vi "cqtDDSdllOpen.vi"   [LabVIEW 2009, in "run.lvlib"]
uses:
  run.lvlib
  C:/Program Files/National Instruments/LabVIEW 2009/instr.lib/CQT_DDS/DDSLibrary/20111109/CQTAD9958.dll
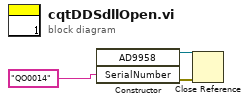
[diagram p0: block diagram]
diagram:
  n1 = constructor class="AD9958"("SerialNumber"="QO0014") -> (reference out=w1:refnum<k24>, error out=w3:errorcluster)  [unwired: 3 in, 2 out]
  n2 = Close Reference(reference=w1, error in (no error)=w3) -> ()  [unwired: 1 out]
